vi "Configure Clock_5782.vi"(8 "error in":errorcluster, 10 "Clock Source":T1(ring), 11 "FPGA VI Reference in":T2) -> (0 "error out":errorcluster, 2 "Configuration Error":bool, 3 "FPGA VI Reference Out":T3)   [LabVIEW 2013]
doc: "This VI configures the clock source for the NI 5772. For execution steps, refer to the comments on the block diagram."
uses:
  FPGAref_5782.ctl
  Config/FPGAref_config.ctl
  <vilib>/rvi/interface/common/niFpgaWaitOnOcc.vi
  <vilib>/Utility/error.llb/Error Cluster From Error Code.vi
  <vilib>/rvi/errors/niLvFpgaAdjustHostInterfaceError.vi
  <vilib>/rvi/interface/nirviReadWriteControl/nirviReadWriteControl.xnode
  <vilib>/rvi/interface/Simulation/niFpgaSimulationCallBeginRW.vi
  NiFpgaLv.dll
panel:
  # "This VI configures the clock source for the NI 5771. For execution steps, refer to the comments on the block diagram."
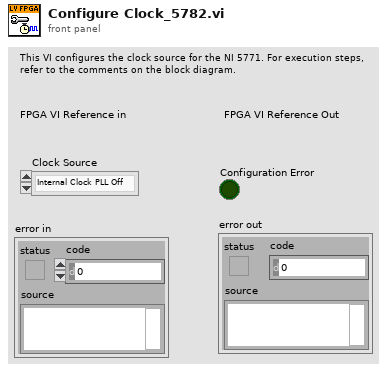
[diagram p1: front panel]
types:
  T1 = enum8{"Internal Clock PLL Off", "Internal Clock PLL On (REF IN)", "External Clock (CLK_IN)", "Internal Clock PLL On (IoModSyncClk)"}
  T2 = typedef "FPGAref_config.ctl" = refnum<k20>
  T3 = typedef "FPGAref_5782.ctl" = refnum<k20>
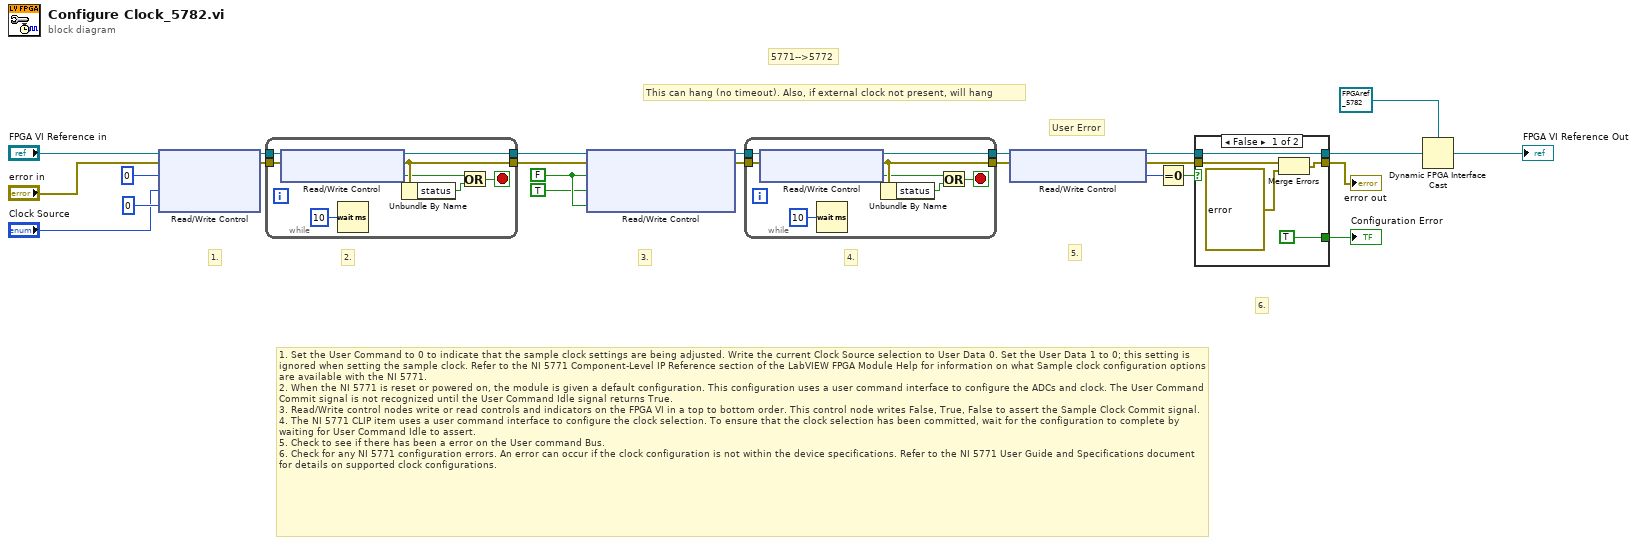
[diagram p0: block diagram]
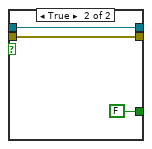
[diagram p2: hidden frame]
diagram:
  w19 = FALSE ("Sample Clock Commit")
  # "User Error"
  # "5771-->5772"
  # "This can hang (no timeout). Also, if external clock not present, will hang"
  # "6."
  # "1. Set the User Command to 0 to indicate that the sample clock settings are being adjusted. Write the current Clock Source selection to User Data 0. Set the User Data 1 to 0; this setting is ignored when setting the sample clock. Refer to the NI 5771 Component-Level IP Reference section of the LabVIEW FPGA Module Help for information on what Sample clock configuration options are available with the NI 5771.\n2. When the NI 5771 is reset or powered on, the module is given a default configuration. This configuration uses a user command interface to configure the ADCs and clock. The User Command Commit signal is not recognized until the User Command Idle signal returns True.\n3. Read/Write control nodes write or read controls and indicators on the FPGA VI in a top to bottom order. This control node writes False, True, False to assert the Sample Clock Commit signal.\n4. The NI 5771 CLIP item uses a user command interface to configure the clock selection. To ensure that the clock selection has been committed, wait for the configuration to complete by waiting for User Command Idle to assert.\n5. Check to see if there has been a error on the User command Bus. \n6. Check for any NI 5771 configuration errors. An error can occur if the clock configuration is not within the device specifications. Refer to the NI 5771 User Guide and Specifications document for details on supported clock configurations."
  # "5."
  # "4."
  # "3."
  # "2."
  # "1."
  n1 = xnode "Read/Write Control"("FPGA VI Reference In"="FPGA VI Reference in", "error in"="error in", "User Command"=u8 0, "User Data 0"="Clock Source", "User Data 1"=u8 0) -> ("FPGA VI Reference Out"=w23:T2, "error out"=w22:errorcluster)
  n2 = while {
    tunnel: w23 -> [w28]
    tunnel: w22 -> [w29]
    tunnel: [w26] -> w20
    tunnel: [w27] -> w21
    stop <- w30 stop-if-true
    n3 = xnode "Read/Write Control"("FPGA VI Reference In"=w28, "error in"=w29) -> ("FPGA VI Reference Out"=w27:T2, "error out"=w26:errorcluster, "User Command Idle"=w25:bool)
    n4 = Wait (ms)(milliseconds to wait=u32 10) -> ()  [unwired: 1 out]
    n5 = Unbundle By Name(w26) -> ("status"=w31:bool)
    n6 = Or(x=w25, y=w31) -> (x .or. y?=w30:bool)
  }
  n7 = xnode "Read/Write Control"("FPGA VI Reference In"=w21, "error in"=w20, "User Command Commit"=w19, "User Command Commit"=TRUE ("Sample Clock Commit"), "User Command Commit"=w19) -> ("FPGA VI Reference Out"=w16:T2, "error out"=w15:errorcluster)
  n8 = while {
    tunnel: w16 -> [w36]
    tunnel: w15 -> [w37]
    tunnel: [w34] -> w14
    tunnel: [w35] -> w13
    stop <- w38 stop-if-true
    n9 = xnode "Read/Write Control"("FPGA VI Reference In"=w36, "error in"=w37) -> ("FPGA VI Reference Out"=w35:T2, "error out"=w34:errorcluster, "User Command Idle"=w33:bool)
    n10 = Wait (ms)(milliseconds to wait=u32 10) -> ()  [unwired: 1 out]
    n11 = Unbundle By Name(w34) -> ("status"=w39:bool)
    n12 = Or(x=w33, y=w39) -> (x .or. y?=w38:bool)
  }
  n13 = xnode "Read/Write Control"("FPGA VI Reference In"=w13, "error in"=w14) -> ("FPGA VI Reference Out"=w6:T2, "error out"=w10:errorcluster, "User Command Status"=w9:u8)
  n14 = Equal To 0?(x=w9) -> (x = 0?=w8:bool)
  n15 = case shown="False" w8 {
    tunnel: [w45 w48] -> w5
    tunnel: w10 -> [w44 w48]
    tunnel: [TRUE ("Configured?") FALSE ("Configured?")] -> w4
    tunnel: w6 -> [w41 w46]
    tunnel: [w41 w46] -> w3
    frame False {
      n16 = Merge Errors(w44, errorcluster {"status"=TRUE, "code"=-8998, "source"="IO Module clock not configured correctly. Please ensure that the desired clock meets the required specifications."} ("error in")) -> (w45:errorcluster)
    }
    frame True {
    }
  }
  "error out" <- w5
  "Configuration Error" <- w4
  n17 = Dynamic FPGA Interface Cast(Session In=T3 refnum ("FPGA VI Reference Out"), Type=w3) -> (Session Out=→"FPGA VI Reference Out":T3)
